vi "List All Azure Containers.vi"() -> ()   [LabVIEW 2015]
doc: "Demonstrates how to list all containers associated with an Azure storage account."
uses:
  Core/Azure Credentials.ctl
  Core/Session/Session.lvclass
  Core/NI_Azure_Core.lvlib
  Blob Storage/NI_Azure_Blob.lvlib
panel:
  in  "Access Key":string
  in  "Storage Account Name":string
  out "Containers":i32(listbox)
  # "Overview: Demonstrates how to list all containers associated with an Azure storage account.\nRequirements: NI Cloud Toolkit for Azure and a registered Microsoft Azure account\nInstructions:\n1. Specify the Storage Account Name and Access Key for your Azure account. You can create an account at http://azure.microsoft.com.\n2. Run the VI. All the containers associated with your account should be listed in the Containers indicator."
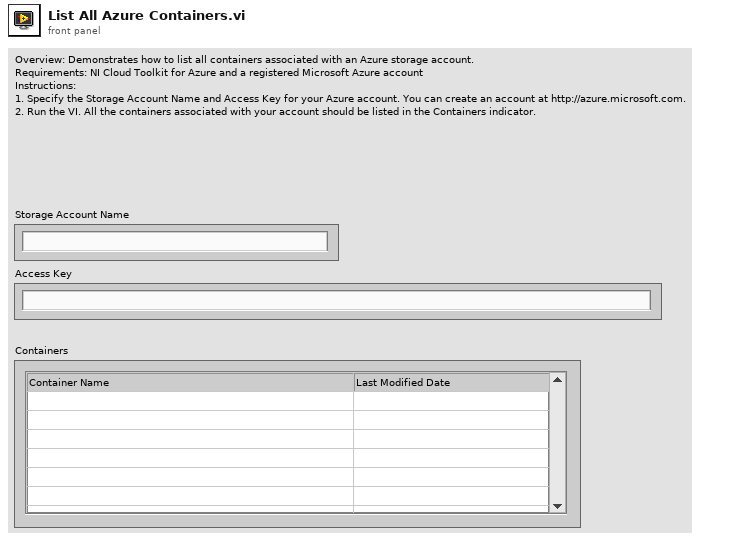
[diagram p1: front panel]
types:
  T1 = typedef "NI_Azure_Core.lvlib/Azure Credentials.ctl" = cluster{"Storage Account Name":string, "Access Key":string}
  T2 = typedef "NI_Azure_Core.lvlib/Name Value Pair.ctl" = cluster{"name":string, "value":string}
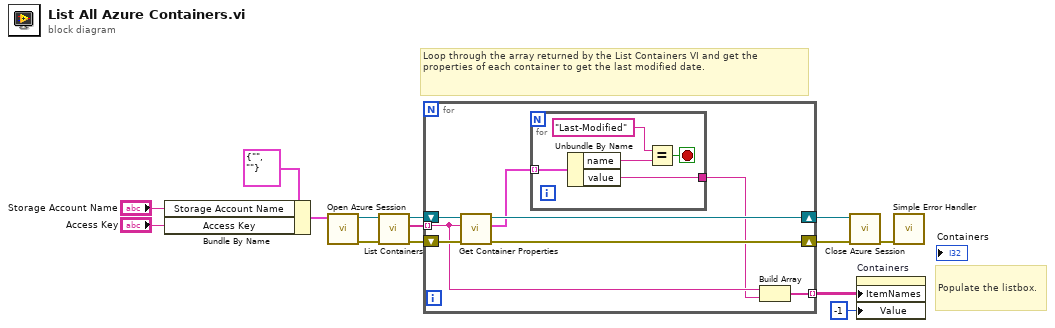
[diagram p0: block diagram]
diagram:
  # "Populate the listbox."
  # "Loop through the array returned by the List Containers VI and get the properties of each container to get the last modified date."
  n1 = Bundle By Name(cluster=T1 {"Storage Account Name"="", "Access Key"=""} ("Credentials"), "Storage Account Name"="Storage Account Name", "Access Key"="Access Key") -> (w12:T1)
  n2 = call "Open Azure Session.vi"("Credentials"=w12) -> ("error out"=w10:errorcluster, "Azure Session"=w9:refnum<class "Session.lvclass">)  [unwired: 9 in]
  n3 = call "List Containers.vi"("error in (no error)"=w10, "Azure Session in"=w9) -> ("error out"=w7:errorcluster, "Containers"=w6:string[], "Azure Session out"=w8:refnum<class "Session.lvclass">)  [unwired: 7 in]
  n4 = for {
    shift-right: [w20] -> w4
    shift-left: w8 -> [w22]
    tunnel: w6 -> [w18] mode=indexing
    shift-right: [w19] -> w5
    shift-left: w7 -> [w21]
    tunnel: [w15] -> w2 mode=indexing
    n5 = call "Get Container Properties.vi"("error in (no error)"=w21, "Container"=w18, "Azure Session in"=w22) -> ("error out"=w19:errorcluster, "Container Properties"=w17:T2[], "Azure Session out"=w20:refnum<class "Session.lvclass">)  [unwired: 6 in]
    n6 = for {
      tunnel: w17 -> [w27] mode=indexing
      tunnel: [w26] -> w16
      stop <- w24 stop-if-true
      n7 = Unbundle By Name(w27) -> ("name"=w25:string, "value"=w26:string)
      n8 = Equal?(x="Last-Modified", y=w25) -> (x = y?=w24:bool)
    }
    n9 = Build Array(w18, w16) -> (w15:string[])
  }
  n10 = call "Close Azure Session.vi"("error in (no error)"=w5, "Azure Session"=w4) -> ("error out"=w3:errorcluster)  [unwired: 9 in]
  n11 = property on="Containers" class="MCListbox (strict)"("ItemNames"=w2, "Value"=-1 ("Containers")) -> ()  [unwired: 2 in, 2 out]
  n12 = call <vilib>:"Simple Error Handler.vi"("error in (no error)"=w3) -> ()  [unwired: 4 in, 5 out]
